vi "Create Evaluations.vi"(8 "error in (no error)":errorcluster, 11 "IEvaluation in":refnum<class "Harmonics_Relative_Power.lvclass">) -> (0 "error out":errorcluster, 2 "Evaluations Out":T1[](array[typedef]) {"Low Limit" format="%#_13g"; "SI Scaling" items=["femto"=-15, "pico"=-12, "nano"=-9, "micro"=-6, "milli"=-3, "percent"=-2, ""=0, "kilo"=3, "mega"=6, "giga"=9, "tera"=12]}, 3 "IEvaluation out":refnum<class "Harmonics_Relative_Power.lvclass">)   [LabVIEW 2016, in "SeqAuto Evaluations.lvlib" / "Harmonics_Relative_Power.lvclass"]
uses:
  Harmonics_Relative_Power.lvclass
  C:/projects/STS/Common/Sequence Automation/Plugins/SeqAuto IEvaluation.lvlibp/SeqAuto IEvaluation.lvclass
  Plugins/TestStand API Tools (TSAT).lvlibp/Evaluation Actions/Includes/Controls/TSAT Evaluation.ctl
  Plugins/TestStand API Tools (TSAT).lvlibp/Evaluation Actions/Includes/Controls/TSAT Eval SI Unit Scaling.ctl
  Plugins/TestStand API Tools (TSAT).lvlibp/Evaluation Actions/Includes/Controls/TSAT Evaluation Type.ctl
  Harmonics_Relative_Power.lvclass/Harmonics_Relative_Power.ctl
  Read Export Data Locations.vi
  Read Harmonics.vi
  Plugins/SeqAuto IEvaluation.lvlibp/Read Measurement Name.vi
  Plugins/TestStand API Tools (TSAT).lvlibp/Evaluation Actions/TSAT Evaluation Actions.lvlib
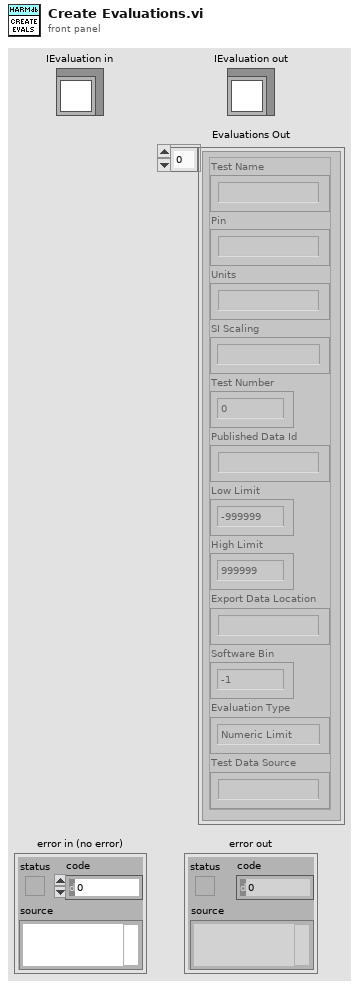
[diagram p1: front panel]
types:
  T1 = typedef "TestStand API Tools (TSAT).lvlibp/TSAT Evaluation Actions.lvlib/TSAT Evaluation.ctl" = cluster{"Test Name":string, "Pin":string, "Units":string, "SI Scaling":T2, "Test Number":i32, "Published Data Id":string, "Low Limit":dbl, "High Limit":dbl, "Export Data Location":string, "Software Bin":i64, "Evaluation Type":T3, "Test Data Source":string}
  T2 = typedef "TestStand API Tools (TSAT).lvlibp/TSAT Evaluation Actions.lvlib/TSAT Eval SI Unit Scaling.ctl" = i16
  T3 = typedef "TestStand API Tools (TSAT).lvlibp/TSAT Evaluation Actions.lvlib/TSAT Evaluation Type.ctl" = enum16{"Numeric Limit", "Pass/Fail", "None"}
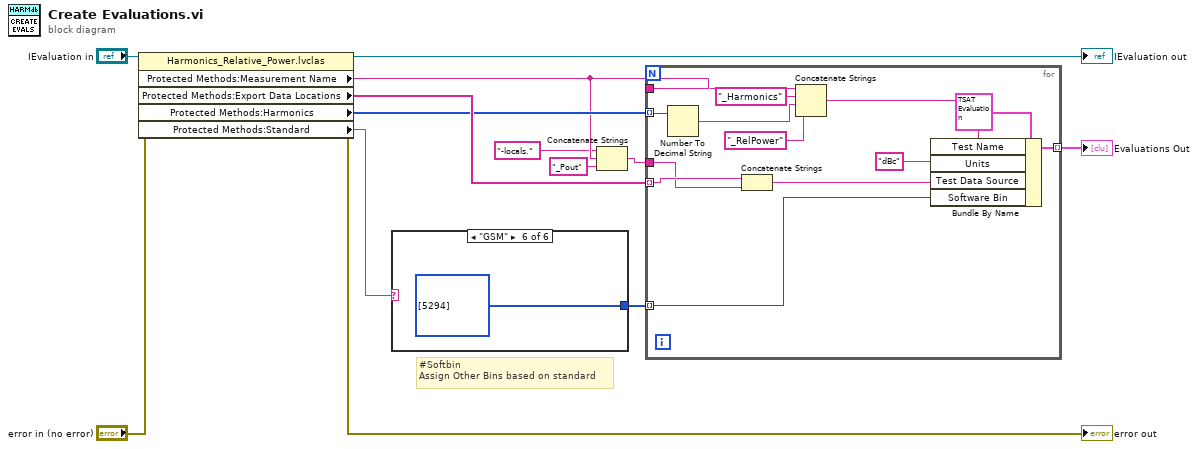
[diagram p0: block diagram]
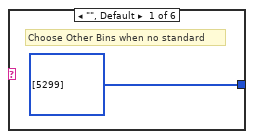
[diagram p2: hidden frame]
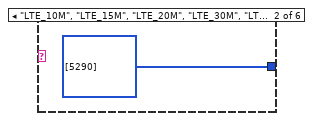
[diagram p3: hidden frame]
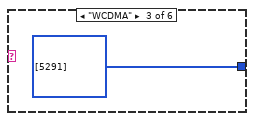
[diagram p4: hidden frame]
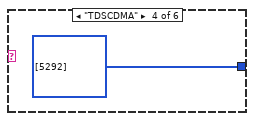
[diagram p5: hidden frame]
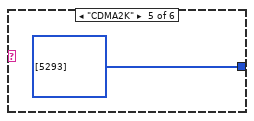
[diagram p6: hidden frame]
diagram:
  # "#Softbin \nAssign Other Bins based on standard"
  n1 = property class="Harmonics_Relative_Power.lvclas"(reference="IEvaluation in", error in="error in (no error)") -> (reference out=→"IEvaluation out":refnum<class "Harmonics_Relative_Power.lvclass">, error out=→"error out":errorcluster, "Protected Methods:Measurement Name"=w4:string, "Protected Methods:Export Data Locations"=w6:string[], "Protected Methods:Harmonics"=w5:i8[], "Protected Methods:Standard"=w2:string)
  n2 = case shown="\"GSM\"" w2 {
    tunnel: [i64[] [5299] i64[] [5290] i64[] [5291] i64[] [5292] i64[] [5293] i64[] [5294]] -> w1
    frame "", Default {
      # "Choose Other Bins when no standard"
    }
    frame "LTE_10M", "LTE_15M", "LTE_20M", "LTE_30M", "LTE_40M" {
    }
    frame "WCDMA" {
    }
    frame "TDSCDMA" {
    }
    frame "CDMA2K" {
    }
    frame "GSM" {
    }
  }
  n3 = Concatenate Strings("-locals." ("string"), w4, "_Pout" ("string")) -> (w7:string)
  n4 = for {
    tunnel: [w31] -> w9 mode=indexing
    tunnel: w7 -> [w21]
    tunnel: w6 -> [w22] mode=indexing
    tunnel: w5 -> [w25] mode=indexing
    tunnel: w4 -> [w28]
    tunnel: w1 -> [w20] mode=indexing
    n5 = Number To Decimal String(number=w25) -> (decimal integer string=w24:string)  [unwired: 1 in]
    n6 = Concatenate Strings(w22, w21) -> (w29:string)
    n7 = Concatenate Strings(w28, "_Harmonics" ("string"), w24, "_RelPower" ("string")) -> (w26:string)
    n8 = Bundle By Name(cluster=T1 {"Test Name"="", "Pin"="", "Units"="", "SI Scaling"=0, "Test Number"=0, "Published Data Id"="", "Low Limit"=-999999.0, "High Limit"=999999.0, "Export Data Location"="", "Software Bin"=-1, "Evaluation Type"=enum."Numeric Limit", "Test Data Source"=""} ("Evaluation"), "Test Name"=w26, "Units"="dBc", "Test Data Source"=w29, "Software Bin"=w20) -> (w31:T1)
  }
  "Evaluations Out" <- w9
